vi "Simulation Settings Global.vi"() -> ()   [LabVIEW 2013]
uses:
  Simulation/Simulation Settings Cluster.ctl
panel:
  in  "Simulation Settings":T1
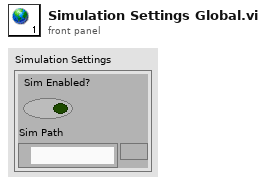
[diagram p1: front panel]
types:
  T1 = typedef "Simulation Settings Cluster.ctl" = cluster{"Sim Enabled?":bool, "Sim Path":path}
diagram:
